vi "FloatToHex.vi"(11 "数组输入":sgl[](array[numeric])) -> (3 "数组":u16[](array[numeric]))   [LabVIEW 2016, in "超标留样集成.lvlib" / "ESTD1200.lvlib"]
uses:
  ESTD1200.lvlib
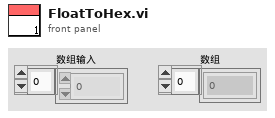
[diagram p1: front panel]
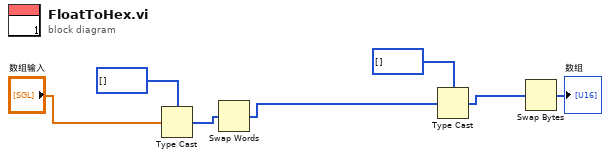
[diagram p0: block diagram]
diagram:
  n1 = Type Cast(type=u32[] [], x="数组输入") -> (*(type *) &x=w3:u32[])
  n2 = Swap Words(1:w3) -> (0:w5:u32[])
  n3 = Type Cast(type=u16[] [], x=w5) -> (*(type *) &x=w6:u16[])
  n4 = Swap Bytes(anything=w6) -> (byte swapped=→"数组":u16[])
